vi "Station Get By sxStationId.vi"(8 "error in (no error)":errorcluster, 10 "sxStationId (\"\")":string, 11 "Connection Refnum":T2) -> (0 "error out":errorcluster, 1 "Instruments on Station":T1[](array[typedef]), 2 "Station Record":T3, 3 "Connection Refnum":T2, 4 "Data Present?":bool)   [LabVIEW 2011]
uses:
  Station Record.ctl
  SI.LIB/ODBC/SQL Controls/Connection Refnum.ctl
  Instruments/Instrument Record.ctl
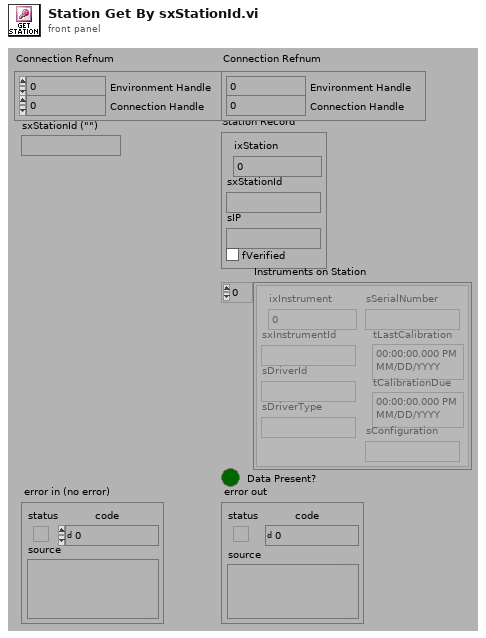
[diagram p1: front panel]
types:
  T1 = typedef "Instrument Record.ctl" = cluster{"ixInstrument":i32, "sxInstrumentId":string, "sDriverId":string, "sDriverType":string, "sSerialNumber":string, "tLastCalibration":timestamp, "tCalibrationDue":timestamp, "sConfiguration":string}
  T2 = typedef "Connection Refnum.ctl" = cluster{"Environment Handle":i32, "Connection Handle":i32}
  T3 = typedef "Station Record.ctl" = cluster{"ixStation":i32, "sxStationId":string, "sIP":string, "fVerified":bool}
  T4 = typedef "Statement Refnum.ctl" = cluster{"Statement Handle":i32, "Parameter Number":u16}
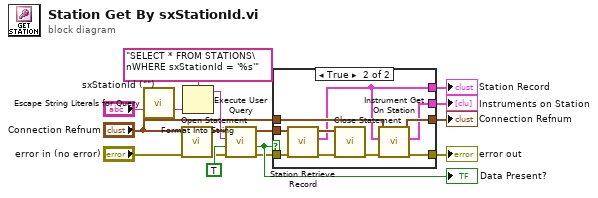
[diagram p0: block diagram]
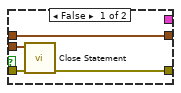
[diagram p2: hidden frame]
diagram:
  n1 = call "Escape String Literals for Query.vi"("String"="sxStationId (\"\")") -> ("escaped String"=w3:string)  [unwired: 1 in, 13 out]
  n2 = call "Open Statement.vi"("error in (no error)"="error in (no error)", "Connection Refnum"="Connection Refnum") -> ("error out"=w12:errorcluster, "Statement Refnum"=w11:T4)  [unwired: 4 out]
  n3 = Format Into String(format string="SELECT * FROM STATIONS\nWHERE sxStationId = '%s'" ("User Query"), w3) -> (resulting string=w10:string)  [unwired: 2 in, 1 out]
  n4 = call "Execute User Query.vi"("error in (no error)"=w12, "Return Data? (f)"=TRUE, "User Query"=w10, "Statement Refnum"=w11) -> ("error out"=w15:errorcluster, "Data Present?"=w16:bool, "Statement Refnum"=w14:T4)  [unwired: 1 out]
  "Data Present?" <- w16
  n5 = case shown="True" w16 {
    tunnel: w15 -> [w19 w30]
    tunnel: w14 -> [w18 w29]
    tunnel: [w17 w25] -> w8
    tunnel: "Connection Refnum" -> [w20 w24]
    tunnel: [w20 w23] -> w7
    tunnel: [_ w22] -> w6
    tunnel: [_ w21] -> w5
    frame False {
      n6 = call "Close Statement.vi"("error in (no error)"=w19, "Statement Refnum"=w18) -> ("error out"=w17:errorcluster)  [unwired: 5 out]
    }
    frame True {
      n7 = call "Station Retrieve Record.vi"("error in (no error)"=w30, "Statement Refnum"=w29) -> ("error out"=w28:errorcluster, "Station Record"=w21:T3, "Statement Refnum"=w27:T4)  [unwired: 7 out]
      n8 = call "Close Statement.vi"("error in (no error)"=w28, "Statement Refnum"=w27) -> ("error out"=w26:errorcluster)  [unwired: 5 out]
      n9 = call "Instrument Get On Station.vi"("error in (no error)"=w26, "Station Record"=w21, "Connection Refnum"=w24) -> ("error out"=w25:errorcluster, "Instruments on Station"=w22:T1[], "Connection Refnum"=w23:T2)  [unwired: 6 out]
    }
  }
  "error out" <- w8
  "Connection Refnum" <- w7
  "Instruments on Station" <- w6
  "Station Record" <- w5
